vi "Init.vi"(8 "error in":errorcluster, 11 "Series Actor in":refnum<class "Series Actor.lvclass">) -> (0 "error out":errorcluster, 1 "Target Virt Instrs":T1(array[cluster]), 2 "Target Physical Instr CFGs":string[](array[string]), 3 "Series Actor out":refnum<class "Series Actor.lvclass">)   [LabVIEW 2024, in "Series Actor.lvlib" / "Series Actor.lvclass"]
uses:
  Series Actor.lvclass
  HAL/MSS/MSS.lvclass
  Series Actor.lvclass/Series Actor.ctl
  2f1605c6-6c78-490f-a4e3-54cad3d2f405.vi
  2f1605c6-6c78-490f-a4e3-54cad3d2f405.vi/a4169a97-72fc-4003-a778-603cf20cafa0.vi
  <vilib>/JDP Science/JSONtext/Find Item.vi
  <vilib>/JDP Science/JSONtext/Next JSON Value.vi
  <vilib>/JDP Science/JSONtext/String Subset.vi
  <vilib>/JDP Science/JSONtext/Parsing/Advance past next JSON Value (inlined COPY).vi
  <vilib>/JDP Science/JSONtext/Parsing/Advance past whitespace.vi
  <vilib>/JDP Science/JSONtext/Parsing/Advance past String.vi
  <vilib>/JDP Science/JSONtext/Parsing/Advance past Number.vi
  <vilib>/JDP Science/JSONtext/Parsing/Advance past Line Ending.vi
  <vilib>/JDP Science/JSONtext/Parsing/Parse Full Path or Item Name.vi
  <vilib>/JDP Science/JSONtext/Parsing/Advance past Array.vi
  <vilib>/JDP Science/JSONtext/Parsing/Advance past Object.vi
  <vilib>/JDP Science/JSONtext/support/Error Cluster From Code.vi
  <vilib>/JDP Science/JSONtext/Offset/Find Item Locations by Path.vi
  <vilib>/JDP Science/JSONtext/JSON text to Variant.vi
  <vilib>/Utility/error.llb/Error Cluster From Error Code.vi
  <vilib>/JDP Science/JSONtext/LVClass Serializer/JSONtext LVClass Serializer.lvclass
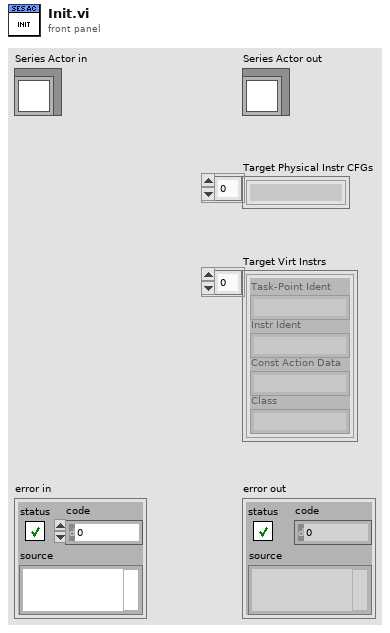
[diagram p1: front panel]
types:
  T1 = cluster{"Task-Point Ident":string, "Instr Ident":string, "Const Action Data":string, "Class":string}[]
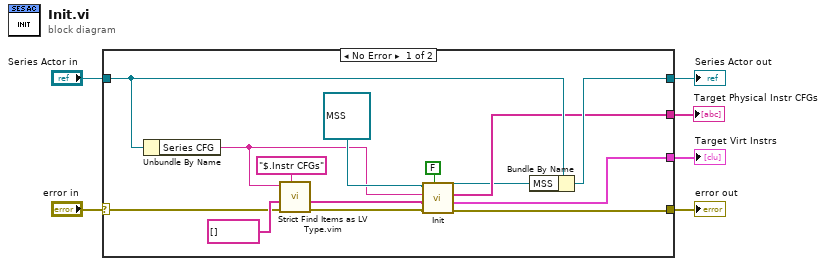
[diagram p0: block diagram]
diagram:
  n1 = case shown="No Error" "error in" {
    selector: "error in" -> [w18 w22]
    tunnel: [w16 w22] -> w5
    tunnel: [w9 w21] -> w3
    tunnel: "Series Actor in" -> [w10 w21]
    tunnel: [w8 _] -> w2
    tunnel: [w11 _] -> w1
    frame No Error {
      n2 = Unbundle By Name(w10) -> ("Series CFG"=w12:string)
      n3 = call "Strict Find Items as LV Type.vim"("$Path or Item Name"="$.Instr CFGs", "error in"=w18, "Data Type and Default Value"=string[] [], "<JSON>"=w12) -> ("error out"=w17:errorcluster, "Data out"=w13:string[])  [unwired: 5 in, 1 out]
      n4 = call "Init.vi"("Is Target?"=FALSE, "error in"=w17, "Instr CFGs"=w13, "<JSON> Virt Instr CFG"=w12, "MSS in"=refnum<class "MSS.lvclass"> refnum ("Host MSS")) -> ("error out"=w16:errorcluster, "Target Virt Instrs"=w11:T1, "Target Instr CFGs"=w8:string[], "MSS out"=w7:refnum<class "MSS.lvclass">)  [unwired: 3 in]
      n5 = Bundle By Name(cluster=w10, "MSS"=w7) -> (w9:refnum<class "Series Actor.lvclass">)
    }
    frame Error {
    }
  }
  "error out" <- w5
  "Series Actor out" <- w3
  "Target Physical Instr CFGs" <- w2
  "Target Virt Instrs" <- w1
